vi "H3C psw cable 28G SFP+读写操作.vi"(6 "input_psw":u8[](array[numeric]) format="%.0x", 7 "input_psw 2":u8[](array[numeric]) format="%.0x", 8 "input_data":u8[](array[numeric]) format="%.0x", 9 "input_mode":string(combo), 10 "Channel":u8 max=5 step=1, 11 "VISA":refnum<visa-resource-name>="COM6") -> (0 "A2Hequal00?":bool, 1 "result":bool, 2 "message":string, 3 "data read":u8[](array[numeric]) format="%.0x")   [LabVIEW 2011]
uses:
  <vilib>/Utility/file.llb/Read From Spreadsheet File (string).vi
panel:
  in  "路径":path
  out "A2h后128个字节":u8[](array[numeric]) format="%.0x"
  out "A2h前128个字节":u8[](array[numeric]) format="%.0x"
  in  "address":u8
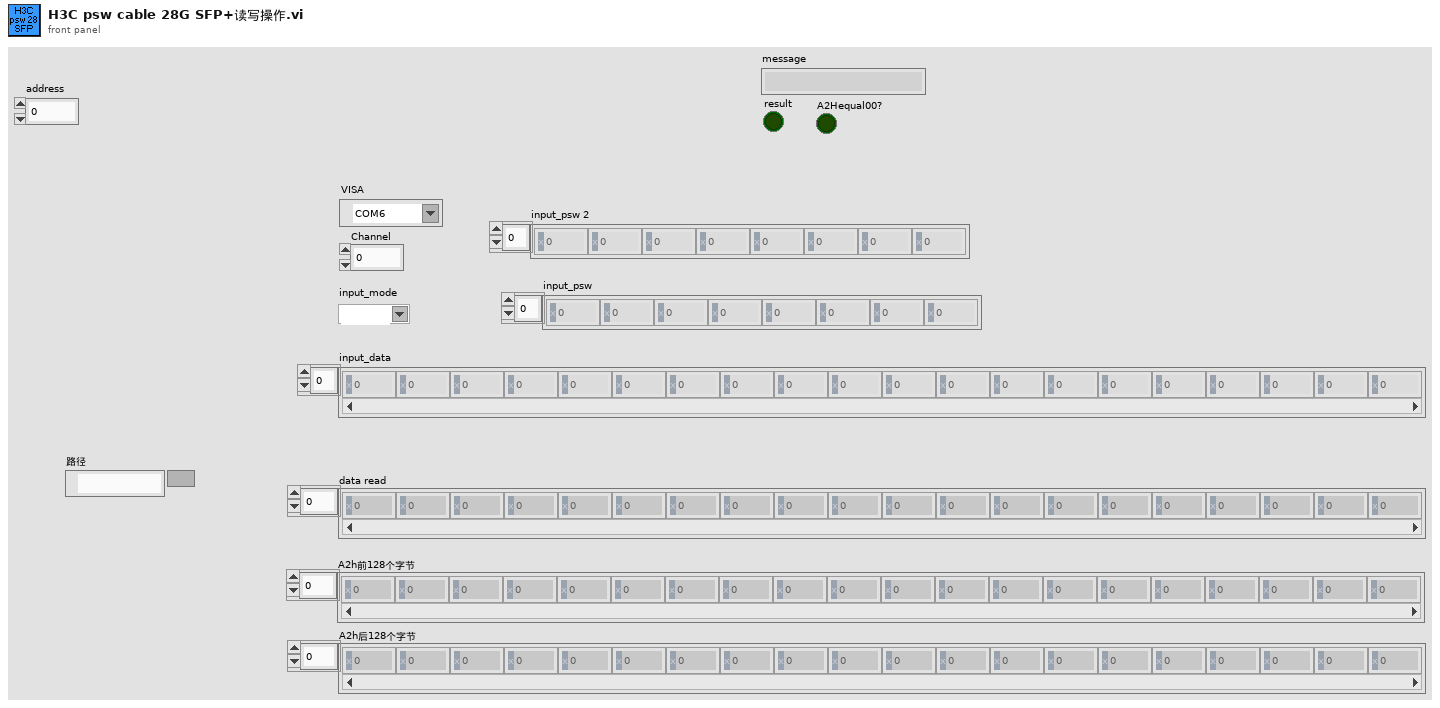
[diagram p1: front panel]
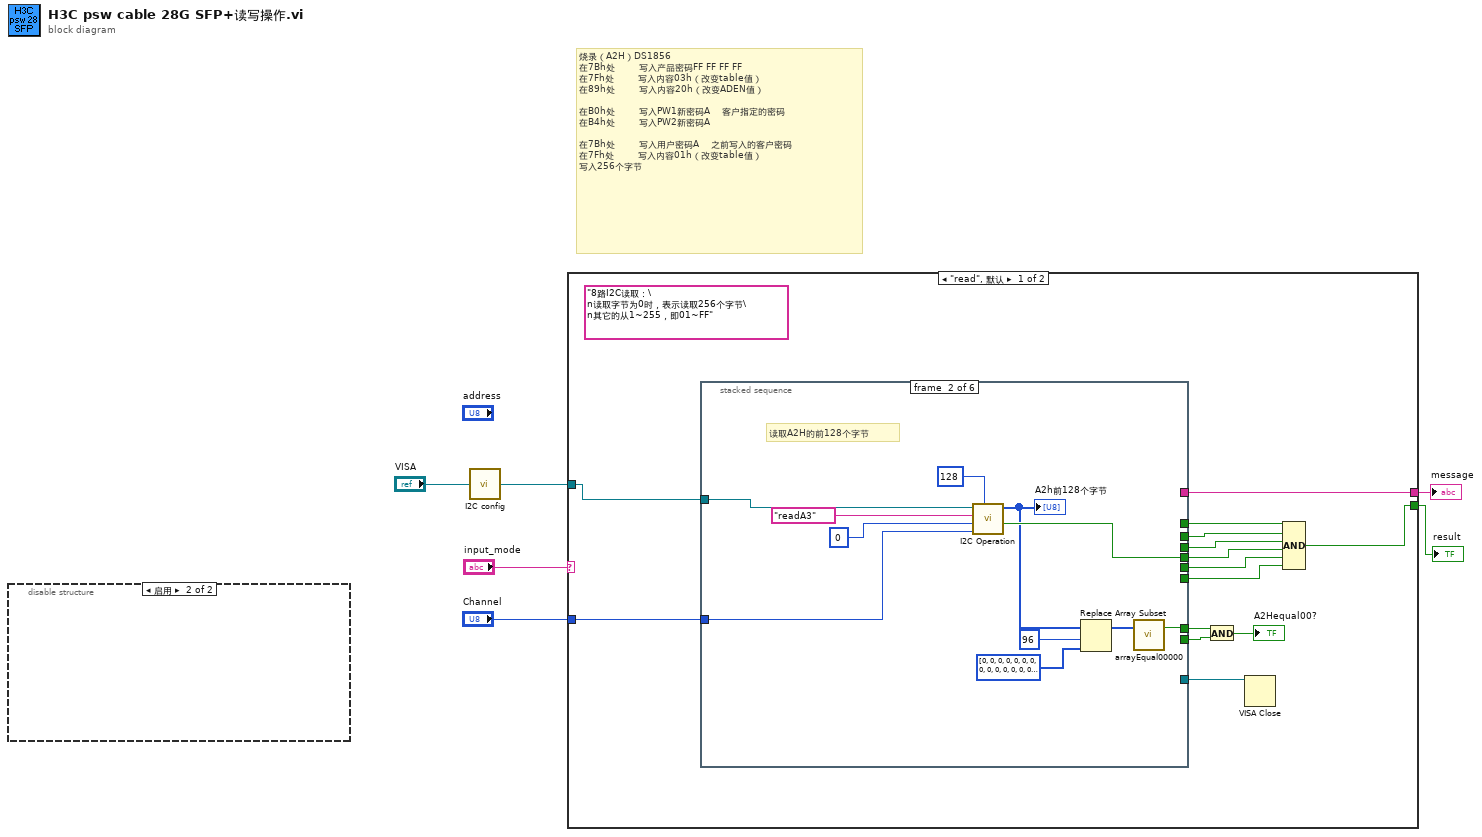
[diagram p0: block diagram]
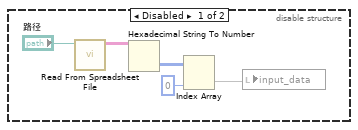
[diagram p2: hidden frame]
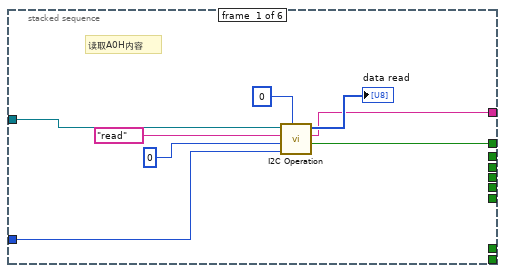
[diagram p3: hidden frame]
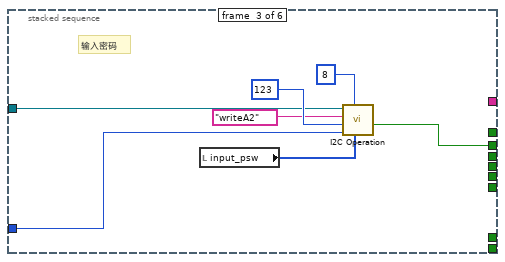
[diagram p4: hidden frame]
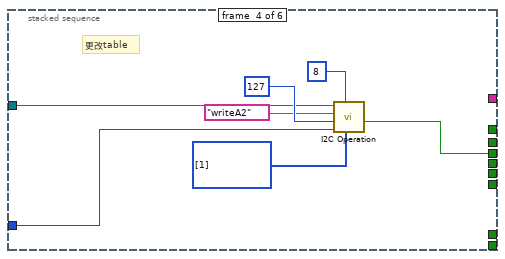
[diagram p5: hidden frame]
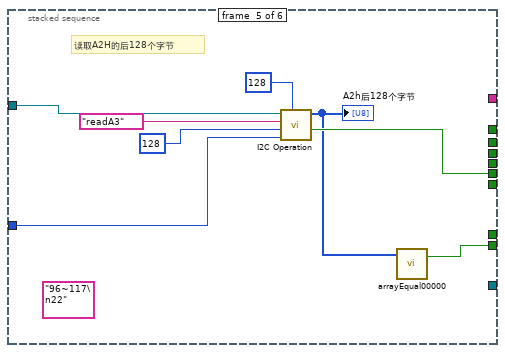
[diagram p6: hidden frame]
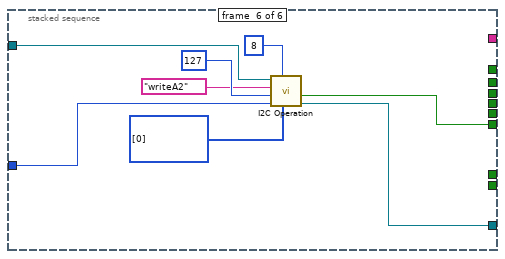
[diagram p7: hidden frame]
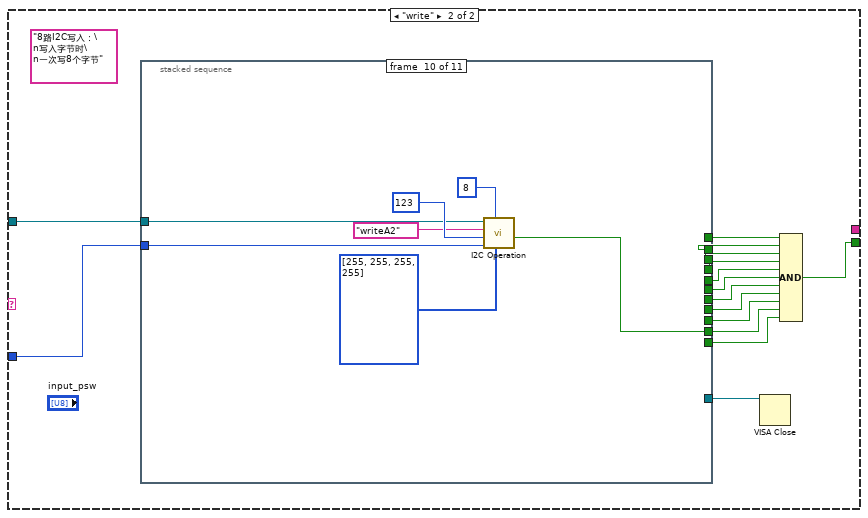
[diagram p8: hidden frame]
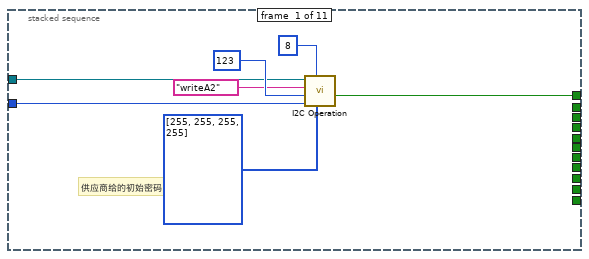
[diagram p9: hidden frame]
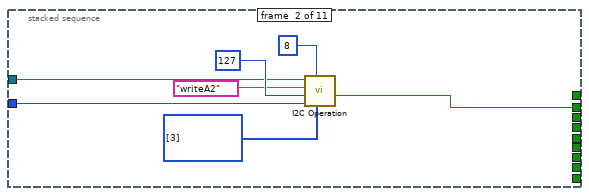
[diagram p10: hidden frame]
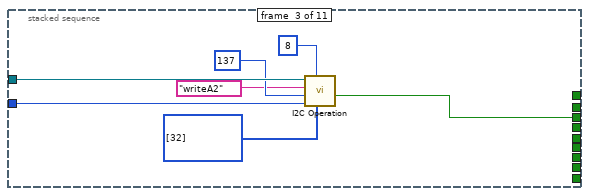
[diagram p11: hidden frame]
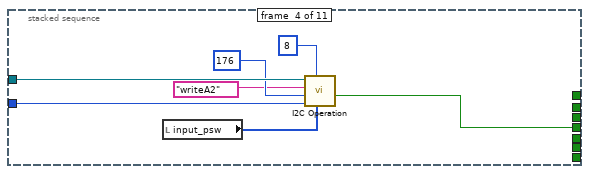
[diagram p12: hidden frame]
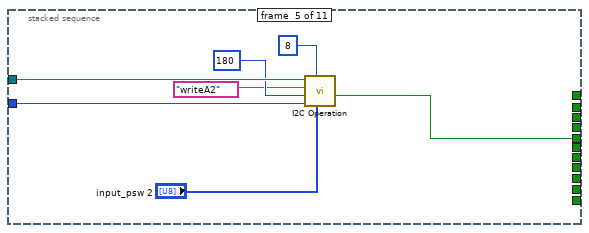
[diagram p13: hidden frame]
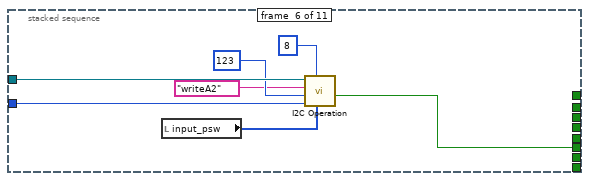
[diagram p14: hidden frame]
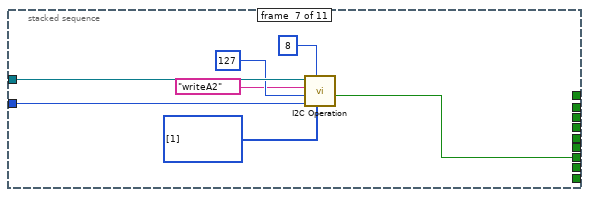
[diagram p15: hidden frame]
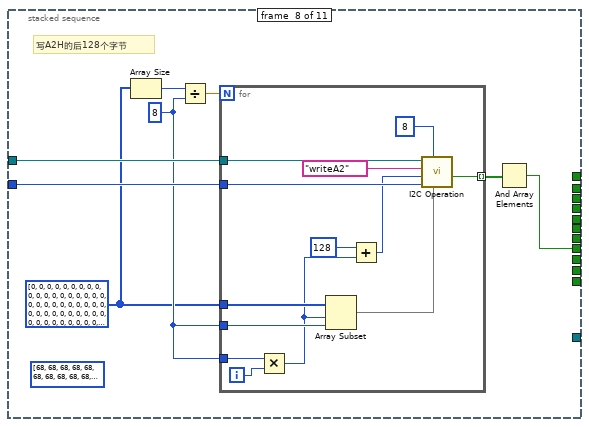
[diagram p16: hidden frame]
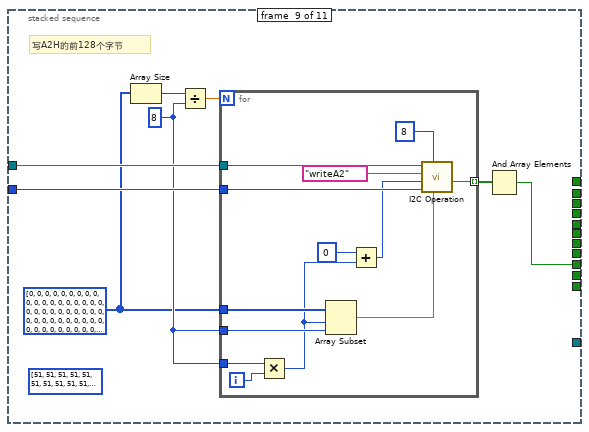
[diagram p17: hidden frame]
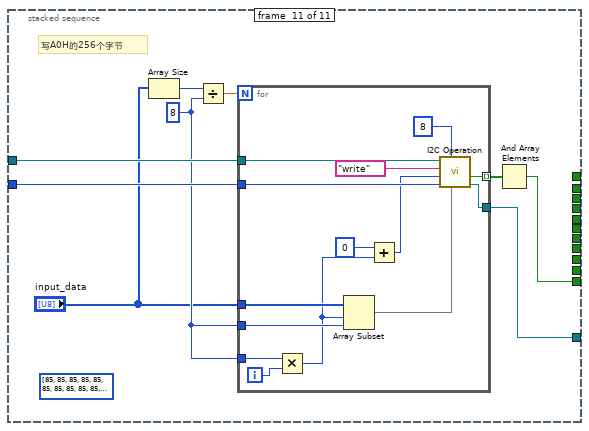
[diagram p18: hidden frame]
diagram:
  # "烧录（A2H）DS1856\n在7Bh处        写入产品密码FF FF FF FF\n在7Fh处        写入内容03h（改变table值）\n在89h处        写入内容20h（改变ADEN值）\n\n在B0h处        写入PW1新密码A    客户指定的密码\n在B4h处        写入PW2新密码A\n\n在7Bh处        写入用户密码A    之前写入的客户密码\n在7Fh处        写入内容01h（改变table值）\n写入256个字节"
  n1 = disable-structure shown="启用" {
    frame Disabled {
      n2 = call-poly <vilib>:"Read From Spreadsheet File.vi"("file path (dialog if empty)"="路径") -> ("all rows"=w10:string[][])  [unwired: 6 in, 4 out]
      n3 = Hexadecimal String To Number(string=w10) -> (number=w9:u32[][])  [unwired: 2 in, 1 out]
      n4 = Index Array(array=w9, index (col)=0 ("禁用的索引 (列)")) -> (element=w7:u32[])  [unwired: 1 in]
      n5 = local write "input_data"(w7) -> ()
    }
    frame Enabled {
    }
  }
  n6 = call "I2C config.vi"("VISA"="VISA") -> ("VISA资源名称输出"=w1:refnum<visa-resource-name>)
  n7 = case shown="\"read\", 默认" "input_mode" {
    tunnel: "Channel" -> [w25 w89]
    tunnel: [w24 _] -> w4
    tunnel: [w18 w77] -> w3
    tunnel: w1 -> [w13 w76]
    frame "read", Default {
      (unwired) "8路I2C读取：\n读取字节为0时，表示读取256个字节\n其它的从1~255，即01~FF"
      n8 = stacked-sequence {
        tunnel: w13 -> [w33 w44 w47 w54 w66 w70]
        tunnel: w25 -> [w30 w41 w46 w53 w63 w69]
        tunnel: [w28 _ _ _ _ _] -> w24
        tunnel: [w27 _ _ _ _ _] -> w23
        tunnel: [_ _ w45 _ _ _] -> w22
        tunnel: [_ _ _ w52 _ _] -> w21
        tunnel: [_ w39 _ _ _ _] -> w20
        tunnel: [_ w38 _ _ _ _] -> w17
        tunnel: [_ _ _ _ w61 _] -> w19
        tunnel: [_ _ _ _ w60 _] -> w16
        tunnel: [_ _ _ _ _ w68] -> w14
        tunnel: [_ _ _ _ _ w67] -> w12
        frame #0 {
          # "读取A0H内容"
          n9 = call "I2C Operation.vi"("size"=0, "Channel"=w30, "address"=u8 0, "mode"="read", "VISA"=w33) -> ("result"=w27:bool, "message"=w28:string, "Data Out"=→"data read":u8[])  [unwired: 3 in, 1 out]
        }
        frame #1 {
          # "读取A2H的前128个字节"
          n10 = call "I2C Operation.vi"("size"=128, "Channel"=w41, "address"=u8 0, "mode"="readA3", "VISA"=w44) -> ("result"=w39:bool, "Data Out"=w34:u8[])  [unwired: 3 in, 2 out]
          "A2h前128个字节" <- w34
          n11 = Replace Array Subset(array=w34, new element=u8[] [0, 0, 0, 0, 0, 0, 0, 0, 0, 0, 0, 0, 0, 0, 0, 0, 0, 0, 0, 0, 0, 0], index=96 ("索引")) -> (w35:u8[])
          n12 = call "arrayEqual00000.vi"("input_array"=w35) -> ("show_bool_result"=w38:bool)  [unwired: 2 in]
        }
        frame #2 {
          # "输入密码"
          n13 = local read "input_psw"() -> (w49:u8[])
          n14 = call "I2C Operation.vi"("input_data"=w49, "size"=8, "Channel"=w46, "address"=u8 123, "mode"="writeA2", "VISA"=w47) -> ("result"=w45:bool)  [unwired: 2 in, 3 out]
        }
        frame #3 {
          # "更改table"
          n15 = call "I2C Operation.vi"("input_data"=u8[] [1], "size"=8, "Channel"=w53, "address"=u8 127, "mode"="writeA2", "VISA"=w54) -> ("result"=w52:bool)  [unwired: 2 in, 3 out]
        }
        frame #4 {
          (unwired) "96~117\n22"
          # "读取A2H的后128个字节"
          n16 = call "I2C Operation.vi"("size"=128, "Channel"=w63, "address"=u8 128, "mode"="readA3", "VISA"=w66) -> ("result"=w61:bool, "Data Out"=w59:u8[])  [unwired: 3 in, 2 out]
          "A2h后128个字节" <- w59
          n17 = call "arrayEqual00000.vi"("input_array"=w59) -> ("show_bool_result"=w60:bool)  [unwired: 2 in]
        }
        frame #5 {
          n18 = call "I2C Operation.vi"("input_data"=u8[] [0], "size"=8, "Channel"=w69, "address"=u8 127, "mode"="writeA2", "VISA"=w70) -> ("VISA  2"=w67:refnum<visa-resource-name>, "result"=w68:bool)  [unwired: 2 in, 2 out]
        }
      }
      n19 = And(x=w17, y=w16) -> (x .and. y?=→"A2Hequal00?":bool)
      n20 = VISA Close(VISA resource name=w12) -> ()  [unwired: 1 in, 1 out]
      n21 = Compound Arithmetic op=AND(w23, w22, w21, w20, w19, w14) -> (w18:bool)
    }
    frame "write" {
      (unwired) "8路I2C写入：\n写入字节时\n一次写8个字节"
      n22 = stacked-sequence {
        tunnel: w76 -> [w90 w97 w110 w117 w124 w131 w138 w146 w167 w184 w196]
        tunnel: w89 -> [w95 w102 w108 w115 w122 w129 w136 w145 w166 w183 w195]
        tunnel: [w91 _ _ _ _ _ _ _ _ _ _] -> w88
        tunnel: [_ w98 _ _ _ _ _ _ _ _ _] -> w87
        tunnel: [_ _ w104 _ _ _ _ _ _ _ _] -> w86
        tunnel: [_ _ _ w111 _ _ _ _ _ _ _] -> w85
        tunnel: [_ _ _ _ w119 _ _ _ _ _ _] -> w84
        tunnel: [_ _ _ _ _ w125 _ _ _ _ _] -> w83
        tunnel: [_ _ _ _ _ _ w132 _ _ _ _] -> w82
        tunnel: [_ _ _ _ _ _ _ w140 _ _ _] -> w81
        tunnel: [_ _ _ _ _ _ _ _ w161 _ _] -> w80
        tunnel: [_ _ _ _ _ _ _ _ _ w181 _] -> w79
        tunnel: [_ _ _ _ _ _ _ _ _ _ w190] -> w78
        tunnel: [_ _ _ _ _ _ _ _ _ _ w188] -> w75
        frame #0 {
          # "供应商给的初始密码"
          n23 = call "I2C Operation.vi"("input_data"=u8[] [255, 255, 255, 255], "size"=8, "Channel"=w95, "address"=u8 123, "mode"="writeA2", "VISA"=w90) -> ("result"=w91:bool)  [unwired: 2 in, 3 out]
        }
        frame #1 {
          n24 = call "I2C Operation.vi"("input_data"=u8[] [3], "size"=8, "Channel"=w102, "address"=u8 127, "mode"="writeA2", "VISA"=w97) -> ("result"=w98:bool)  [unwired: 2 in, 3 out]
        }
        frame #2 {
          n25 = call "I2C Operation.vi"("input_data"=u8[] [32], "size"=8, "Channel"=w108, "address"=u8 137, "mode"="writeA2", "VISA"=w110) -> ("result"=w104:bool)  [unwired: 2 in, 3 out]
        }
        frame #3 {
          n26 = local read "input_psw"() -> (w113:u8[])
          n27 = call "I2C Operation.vi"("input_data"=w113, "size"=8, "Channel"=w115, "address"=u8 176, "mode"="writeA2", "VISA"=w117) -> ("result"=w111:bool)  [unwired: 2 in, 3 out]
        }
        frame #4 {
          n28 = call "I2C Operation.vi"("input_data"="input_psw 2", "size"=8, "Channel"=w122, "address"=u8 180, "mode"="writeA2", "VISA"=w124) -> ("result"=w119:bool)  [unwired: 2 in, 3 out]
        }
        frame #5 {
          n29 = local read "input_psw"() -> (w127:u8[])
          n30 = call "I2C Operation.vi"("input_data"=w127, "size"=8, "Channel"=w129, "address"=u8 123, "mode"="writeA2", "VISA"=w131) -> ("result"=w125:bool)  [unwired: 2 in, 3 out]
        }
        frame #6 {
          n31 = call "I2C Operation.vi"("input_data"=u8[] [1], "size"=8, "Channel"=w136, "address"=u8 127, "mode"="writeA2", "VISA"=w138) -> ("result"=w132:bool)  [unwired: 2 in, 3 out]
        }
        frame #7 {
          (unwired) i32[] [68, 68, 68, 68, 68, 68, 68, 68, 68, 68, 68, 68, 68, 68, 68, 68, 68, 68, 68, 68, 68, 68, 68, 68, 68, 68, 68, 68, 68, 68, 68, 68, 68, 68, 68, 68, 68, 68, 68, 68, 68, 68, 68, 68, 68, 68, 68, 68, 68, 68, 68, 68, 68, 68, 68, 68, 68, 68, 68, 68, 68, 68, 68, 68, 68, 68, 68, 68, 68, 68, 68, 68, 68, 68, 68, 68, 68, 68, 68, 68, 68, 68, 68, 68, 68, 68, 68, 68, 68, 68, 68, 68, 68, 68, 68, 68, 68, 68, 68, 68, 68, 68, 68, 68, 68, 68, 68, 68, 68, 68, 68, 68, 68, 68, 68, 68, 68, 68, 68, 68, 68, 68, 68, 68, 68, 68, 68, 68]
          w142 = 8 ("y")
          w139 = u8[] [0, 0, 0, 0, 0, 0, 0, 0, 0, 0, 0, 0, 0, 0, 0, 0, 0, 0, 0, 0, 0, 0, 0, 0, 0, 0, 0, 0, 0, 0, 0, 0, 0, 0, 0, 0, 0, 0, 0, 0, 0, 0, 0, 0, 0, 0, 0, 0, 0, 0, 0, 0, 0, 0, 0, 0, 0, 0, 0, 0, 0, 0, 0, 0, 0, 0, 0, 0, 0, 0, 0, 0, 0, 0, 0, 0, 0, 0, 0, 0, 0, 0, 0, 0, 0, 0, 0, 0, 0, 0, 0, 0, 0, 0, 0, 0, 0, 0, 0, 0, 0, 0, 0, 0, 0, 0, 0, 0, 0, 0, 0, 0, 0, 0, 0, 0, 0, 0, 0, 0, 0, 0, 0, 0, 0, 0, 0, 0]
          # "写A2H的后128个字节"
          n32 = Array Size(array=w139) -> (size(s)=w144:i32)
          n33 = Divide(x=w144, y=w142) -> (x/y=w143:dbl)
          n34 = for {
            N: w143 -> [_]
            tunnel: w146 -> [w159]
            tunnel: w145 -> [w157]
            tunnel: w139 -> [w155]
            tunnel: w142 -> [w153]
            tunnel: w142 -> [w152]
            tunnel: [w147] -> w141 mode=indexing
            i -> [w154]
            n35 = Multiply(x=w153, y=w154) -> (x*y=w150:i32)
            n36 = Array Subset(array=w155, index=w150, length=w152) -> (w148:u8[])
            n37 = Add(x=u8 128 ("address"), y=w150) -> (x+y=w149:i32)
            n38 = call "I2C Operation.vi"("input_data"=w148, "size"=8, "Channel"=w157, "address"=w149, "mode"="writeA2", "VISA"=w159) -> ("result"=w147:bool)  [unwired: 2 in, 3 out]
          }
          n39 = And Array Elements(Boolean array=w141) -> (logical AND=w140:bool)
        }
        frame #8 {
          (unwired) i32[] [51, 51, 51, 51, 51, 51, 51, 51, 51, 51, 51, 51, 51, 51, 51, 51, 51, 51, 51, 51, 51, 51, 51, 51, 51, 51, 51, 51, 51, 51, 51, 51, 51, 51, 51, 51, 51, 51, 51, 51, 51, 51, 51, 51, 51, 51, 51, 51, 51, 51, 51, 51, 51, 51, 51, 51, 51, 51, 51, 51, 51, 51, 51, 51, 51, 51, 51, 51, 51, 51, 51, 51, 51, 51, 51, 51, 51, 51, 51, 51, 51, 51, 51, 51, 51, 51, 51, 51, 51, 51, 51, 51, 51, 51, 51, 51, 51, 51, 51, 51, 51, 51, 51, 51, 51, 51, 51, 51, 51, 51, 51, 51, 51, 51, 51, 51, 51, 51, 51, 51, 51, 51, 51, 51, 51, 51, 51, 51]
          w163 = 8 ("y")
          w160 = u8[] [0, 0, 0, 0, 0, 0, 0, 0, 0, 0, 0, 0, 0, 0, 0, 0, 0, 0, 0, 0, 0, 0, 0, 0, 0, 0, 0, 0, 0, 0, 0, 0, 0, 0, 0, 0, 0, 0, 0, 0, 0, 0, 0, 0, 0, 0, 0, 0, 0, 0, 0, 0, 0, 0, 0, 0, 0, 0, 0, 0, 0, 0, 0, 0, 0, 0, 0, 0, 0, 0, 0, 0, 0, 0, 0, 0, 0, 0, 0, 0, 0, 0, 0, 0, 0, 0, 0, 0, 0, 0, 0, 0, 0, 0, 0, 0, 0, 0, 0, 0, 0, 0, 0, 0, 0, 0, 0, 0, 0, 0, 0, 0, 0, 0, 0, 0, 0, 0, 0, 0, 0, 0, 0, 0, 0, 0, 0, 0]
          # "写A2H的前128个字节"
          n40 = Array Size(array=w160) -> (size(s)=w165:i32)
          n41 = Divide(x=w165, y=w163) -> (x/y=w164:dbl)
          n42 = for {
            N: w164 -> [_]
            tunnel: w167 -> [w180]
            tunnel: w166 -> [w178]
            tunnel: w160 -> [w176]
            tunnel: w163 -> [w174]
            tunnel: w163 -> [w173]
            tunnel: [w168] -> w162 mode=indexing
            i -> [w175]
            n43 = Multiply(x=w174, y=w175) -> (x*y=w171:i32)
            n44 = Array Subset(array=w176, index=w171, length=w173) -> (w169:u8[])
            n45 = Add(x=u8 0 ("address"), y=w171) -> (x+y=w170:i32)
            n46 = call "I2C Operation.vi"("input_data"=w169, "size"=8, "Channel"=w178, "address"=w170, "mode"="writeA2", "VISA"=w180) -> ("result"=w168:bool)  [unwired: 2 in, 3 out]
          }
          n47 = And Array Elements(Boolean array=w162) -> (logical AND=w161:bool)
        }
        frame #9 {
          n48 = call "I2C Operation.vi"("input_data"=u8[] [255, 255, 255, 255], "size"=8, "Channel"=w183, "address"=u8 123, "mode"="writeA2", "VISA"=w184) -> ("result"=w181:bool)  [unwired: 2 in, 3 out]
        }
        frame #10 {
          (unwired) i32[] [85, 85, 85, 85, 85, 85, 85, 85, 85, 85, 85, 85, 85, 85, 85, 85, 85, 85, 85, 85, 85, 85, 85, 85, 85, 85, 85, 85, 85, 85, 85, 85, 85, 85, 85, 85, 85, 85, 85, 85, 85, 85, 85, 85, 85, 85, 85, 85, 85, 85, 85, 85, 85, 85, 85, 85, 85, 85, 85, 85, 85, 85, 85, 85, 85, 85, 85, 85, 85, 85, 85, 85, 85, 85, 85, 85, 85, 85, 85, 85, 85, 85, 85, 85, 85, 85, 85, 85, 85, 85, 85, 85, 85, 85, 85, 85, 85, 85, 85, 85, 85, 85, 85, 85, 85, 85, 85, 85, 85, 85, 85, 85, 85, 85, 85, 85, 85, 85, 85, 85, 85, 85, 85, 85, 85, 85, 85, 85, 85, 85, 85, 85, 85, 85, 85, 85, 85, 85, 85, 85, 85, 85, 85, 85, 85, 85, 85, 85, 85, 85, 85, 85, 85, 85, 85, 85, 85, 85, 85, 85, 85, 85, 85, 85, 85, 85, 85, 85, 85, 85, 85, 85, 85, 85, 85, 85, 85, 85, 85, 85, 85, 85, 85, 85, 85, 85, 85, 85, 85, 85, 85, 85, 85, 85, 85, 85, 85, 85, 85, 85, 85, 85, 85, 85, 85, 85, 85, 85, 85, 85, 85, 85, 85, 85, 85, 85, 85, 85, 85, 85, 85, 85, 85, 85, 85, 85, 85, 85, 85, 85, 85, 85, 85, 85, 85, 85, 85, 85, 85, 85, 85, 85, 85, 85, 85, 85, 85, 85, 85, 85, 85, 85, 85, 85, 85, 85]
          w192 = 8 ("y")
          # "写A0H的256个字节"
          n49 = Array Size(array="input_data") -> (size(s)=w194:i32)
          n50 = Divide(x=w194, y=w192) -> (x/y=w193:dbl)
          n51 = for {
            N: w193 -> [_]
            tunnel: w196 -> [w210]
            tunnel: w195 -> [w208]
            tunnel: "input_data" -> [w206]
            tunnel: w192 -> [w204]
            tunnel: w192 -> [w203]
            tunnel: [w198] -> w191 mode=indexing
            tunnel: [w197] -> w188
            i -> [w205]
            n52 = Multiply(x=w204, y=w205) -> (x*y=w201:i32)
            n53 = Array Subset(array=w206, index=w201, length=w203) -> (w199:u8[])
            n54 = Add(x=u8 0 ("address"), y=w201) -> (x+y=w200:i32)
            n55 = call "I2C Operation.vi"("input_data"=w199, "size"=8, "Channel"=w208, "address"=w200, "mode"="write", "VISA"=w210) -> ("VISA  2"=w197:refnum<visa-resource-name>, "result"=w198:bool)  [unwired: 2 in, 2 out]
          }
          n56 = And Array Elements(Boolean array=w191) -> (logical AND=w190:bool)
        }
      }
      n57 = VISA Close(VISA resource name=w75) -> ()  [unwired: 1 in, 1 out]
      n58 = Compound Arithmetic op=AND(w88, w87, w86, w85, w84, w83, w82, w81, w80, w79, w78) -> (w77:bool)
    }
  }
  "message" <- w4
  "result" <- w3
